vi "Pert.vi"   [LabVIEW 2013]
uses:
  <vilib>/imath/engines/lvmath2/RunTimeEngine/ErrorHandling/NIMS_Finalize Error.vi
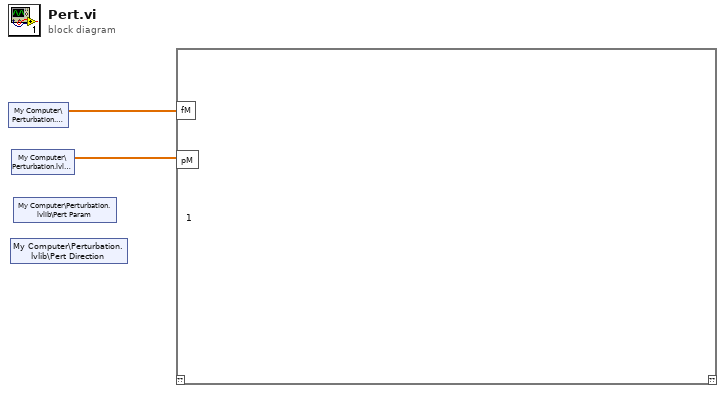
[diagram p0: block diagram]
diagram:
  n1 = shared-variable "My Computer\\Perturbation.lvlib\\fM"() -> (w2:dbl[])  [unwired: 1 in, 1 out]
  n2 = shared-variable "My Computer\\Perturbation.lvlib\\Pert Direction"() -> ()  [unwired: 1 in, 2 out]
  n3 = shared-variable "My Computer\\Perturbation.lvlib\\pM"() -> (w1:dbl[])  [unwired: 1 in, 1 out]
  n4 = shared-variable "My Computer\\Perturbation.lvlib\\Pert Param"() -> ()  [unwired: 1 in, 2 out]
  n5 = mathscript code="1"("fM"=w2, "pM"=w1) -> ()  [unwired: 1 in, 1 out]
